vi "Pos_Calculate Position from distance.vi"(7 "Space size":u32=32, 8 "Error":errorcluster, 11 "Distance":u32) -> (0 "Error Out":errorcluster, 1 "Far Position Out":i32, 2 "Center Position Out":i32, 3 "Near Positoin Out":i32)   [LabVIEW 2024]
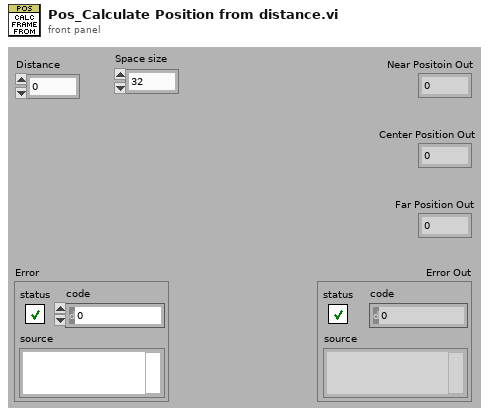
[diagram p1: front panel]
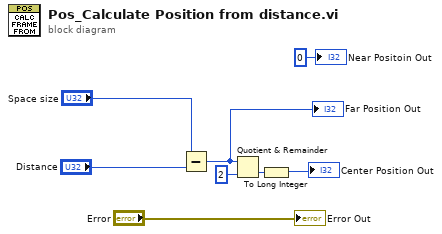
[diagram p0: block diagram]
diagram:
  n1 = Subtract(x="Space size", y="Distance") -> (x-y=w2:u32)
  "Far Position Out" <- w2
  n2 = Quotient & Remainder(x=w2, y=u32 2) -> (floor(x/y)=w6:u32)  [unwired: 1 out]
  n3 = To Long Integer(number=w6) -> (32bit integer=→"Center Position Out":i32)
  "Near Positoin Out" <- 0 ("Near Positoin Out")
  "Error Out" <- "Error"
